vi "메인.vi"() -> ()   [LabVIEW 2021]
uses:
  ctl/AI.ctl
  ctl/RS232.ctl
  ctl/DB.ctl
  ctl/sm.ctl
  ctl/CNN.ctl
  <vilib>/userDefined/High Color/IMAQdx.ctl
  <vilib>/Utility/sysdir.llb/System Directory Type.ctl
  <vilib>/DAQmx/read.llb/DAQmx Read (Analog 1D Wfm NChan NSamp).vi
  <vilib>/Analysis/baseanly.llb/Mean (DBL).vi
  <vilib>/Utility/file.llb/Write Delimited Spreadsheet (DBL).vi
  <vilib>/addons/database/Connection.llb/DB Tools Open Connec (String).vi
  <vilib>/Instr/_visa.llb/VISA Configure Serial Port (Instr).vi
  <vilib>/DAQmx/create/channels.llb/DAQmx Create Channel (AI-Voltage-Basic).vi
  <vilib>/DAQmx/configure/timing.llb/DAQmx Timing (Sample Clock).vi
  <vilib>/DAQmx/miscellaneous.llb/DAQmx Fill In Error Info.vi
  <vilib>/Analysis/NI_AALBase.lvlib
  <vilib>/vision/driver/NI_Vision_Acquisition_Software.lvlib
  <vilib>/addons/database/NI_Database_API.lvlib
panel:
  out "CNN Result":string[](array[string])
  out "Factory 상태":string
  in  "여러 열 리스트박스 2":i32(listbox)
  in  "여러 열 리스트박스":i32(listbox)
  out "Image":T1(plugin-control)
  out "온도":u32[](array[numeric])
  out "배열":dbl[](array[numeric])
  out "거리 센서":waveform(dbl)(graph)
  out "기울기 그래프":waveform(dbl)[](graph)
  out "가속도 그래프":waveform(dbl)(graph)
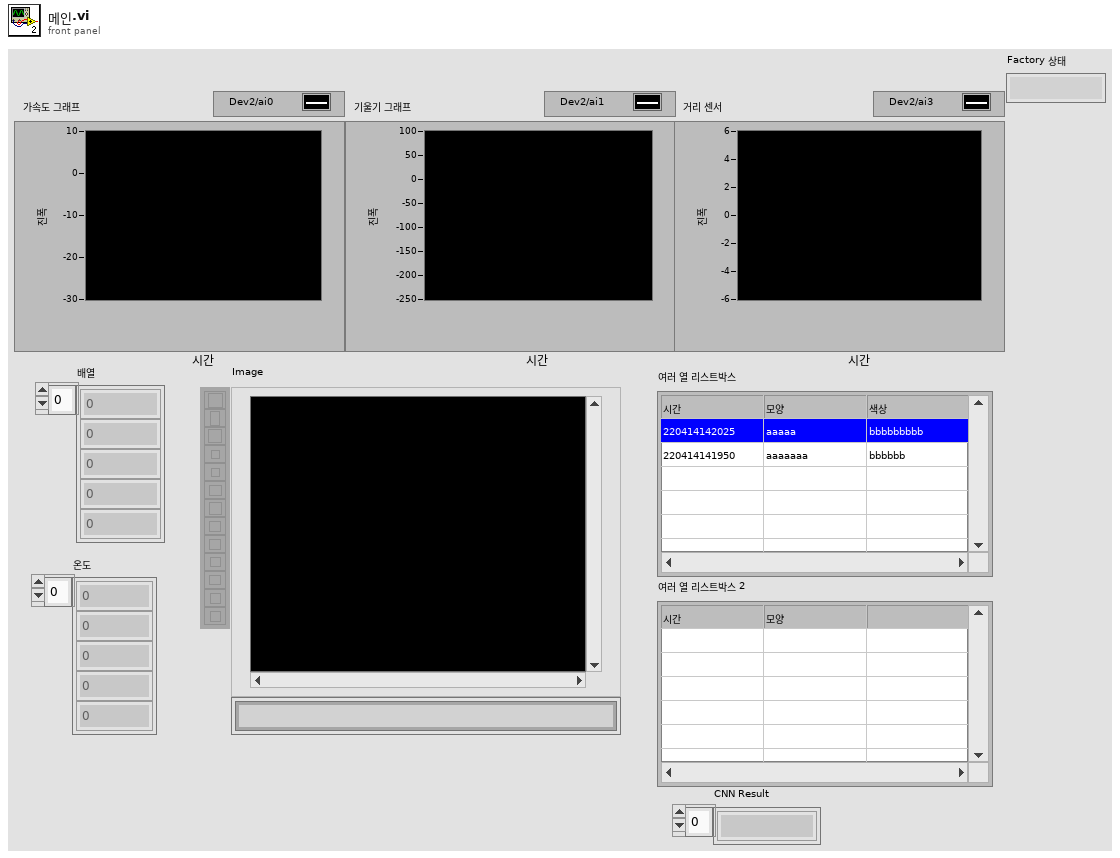
[diagram p1: front panel]
types:
  T1 = typedef "IMAQ Image.ctl" = refnum<image>
  T2 = typedef "비전.ctl" = cluster{"상태":enum16{"초기화", "설정", "상시읽기", "트리거읽기", "닫기", "프로그램정지"}, "값":variant}
  T3 = typedef "CNN.ctl" = cluster{"상태":enum16{"CNN 통신", "프로그램정지"}, "값":variant}
  T4 = typedef "sm.ctl" = cluster{"상태":enum16{"SM통신", "프로그램정지"}, "값":variant}
  T5 = cluster{"메인":refnum<queue>, "AI":refnum<queue>, "RS-232":refnum<queue>, "SM":refnum<queue>, "CNN":refnum<queue>, "DB":refnum<queue>, "비전":refnum<queue>}
  T6 = typedef "메인.ctl" = cluster{"상태":enum16{"초기화", "프로그램정지"}, "값":variant}
  T7 = typedef "DB.ctl" = cluster{"상태":enum16{"초기화", "설정", "값 쓰기", "에러 쓰기", "닫기", "프로그램 정지"}, "값":variant}
  T8 = typedef "RS232.ctl" = cluster{"상태":enum16{"초기화", "설정", "읽기", "닫기", "프로그램정지"}, "값":variant}
  T9 = typedef "AI.ctl" = cluster{"상태":enum16{"초기화", "설정", "읽기", "닫기", "프로그램정지"}, "값":variant}
  T10 = enum16{"초기화", "설정", "값 쓰기", "에러 쓰기", "닫기", "프로그램 정지"}
  T11 = typedef "NI_Database_API.lvlib/Conn ObjectReference.ctl" = refnum<k1>
  T12 = cluster{"[0]":string, "[1]":string, "[2]":string}
  T13 = typedef "IMAQdx.ctl" = refnum<k21>
  T14 = enum16{"초기화", "설정", "상시읽기", "트리거읽기", "닫기", "프로그램정지"}
  T15 = typedef "System Directory Type.ctl" = i32
  T16 = enum16{"Standard", "Buffered", "CRLF", "Immediate"}
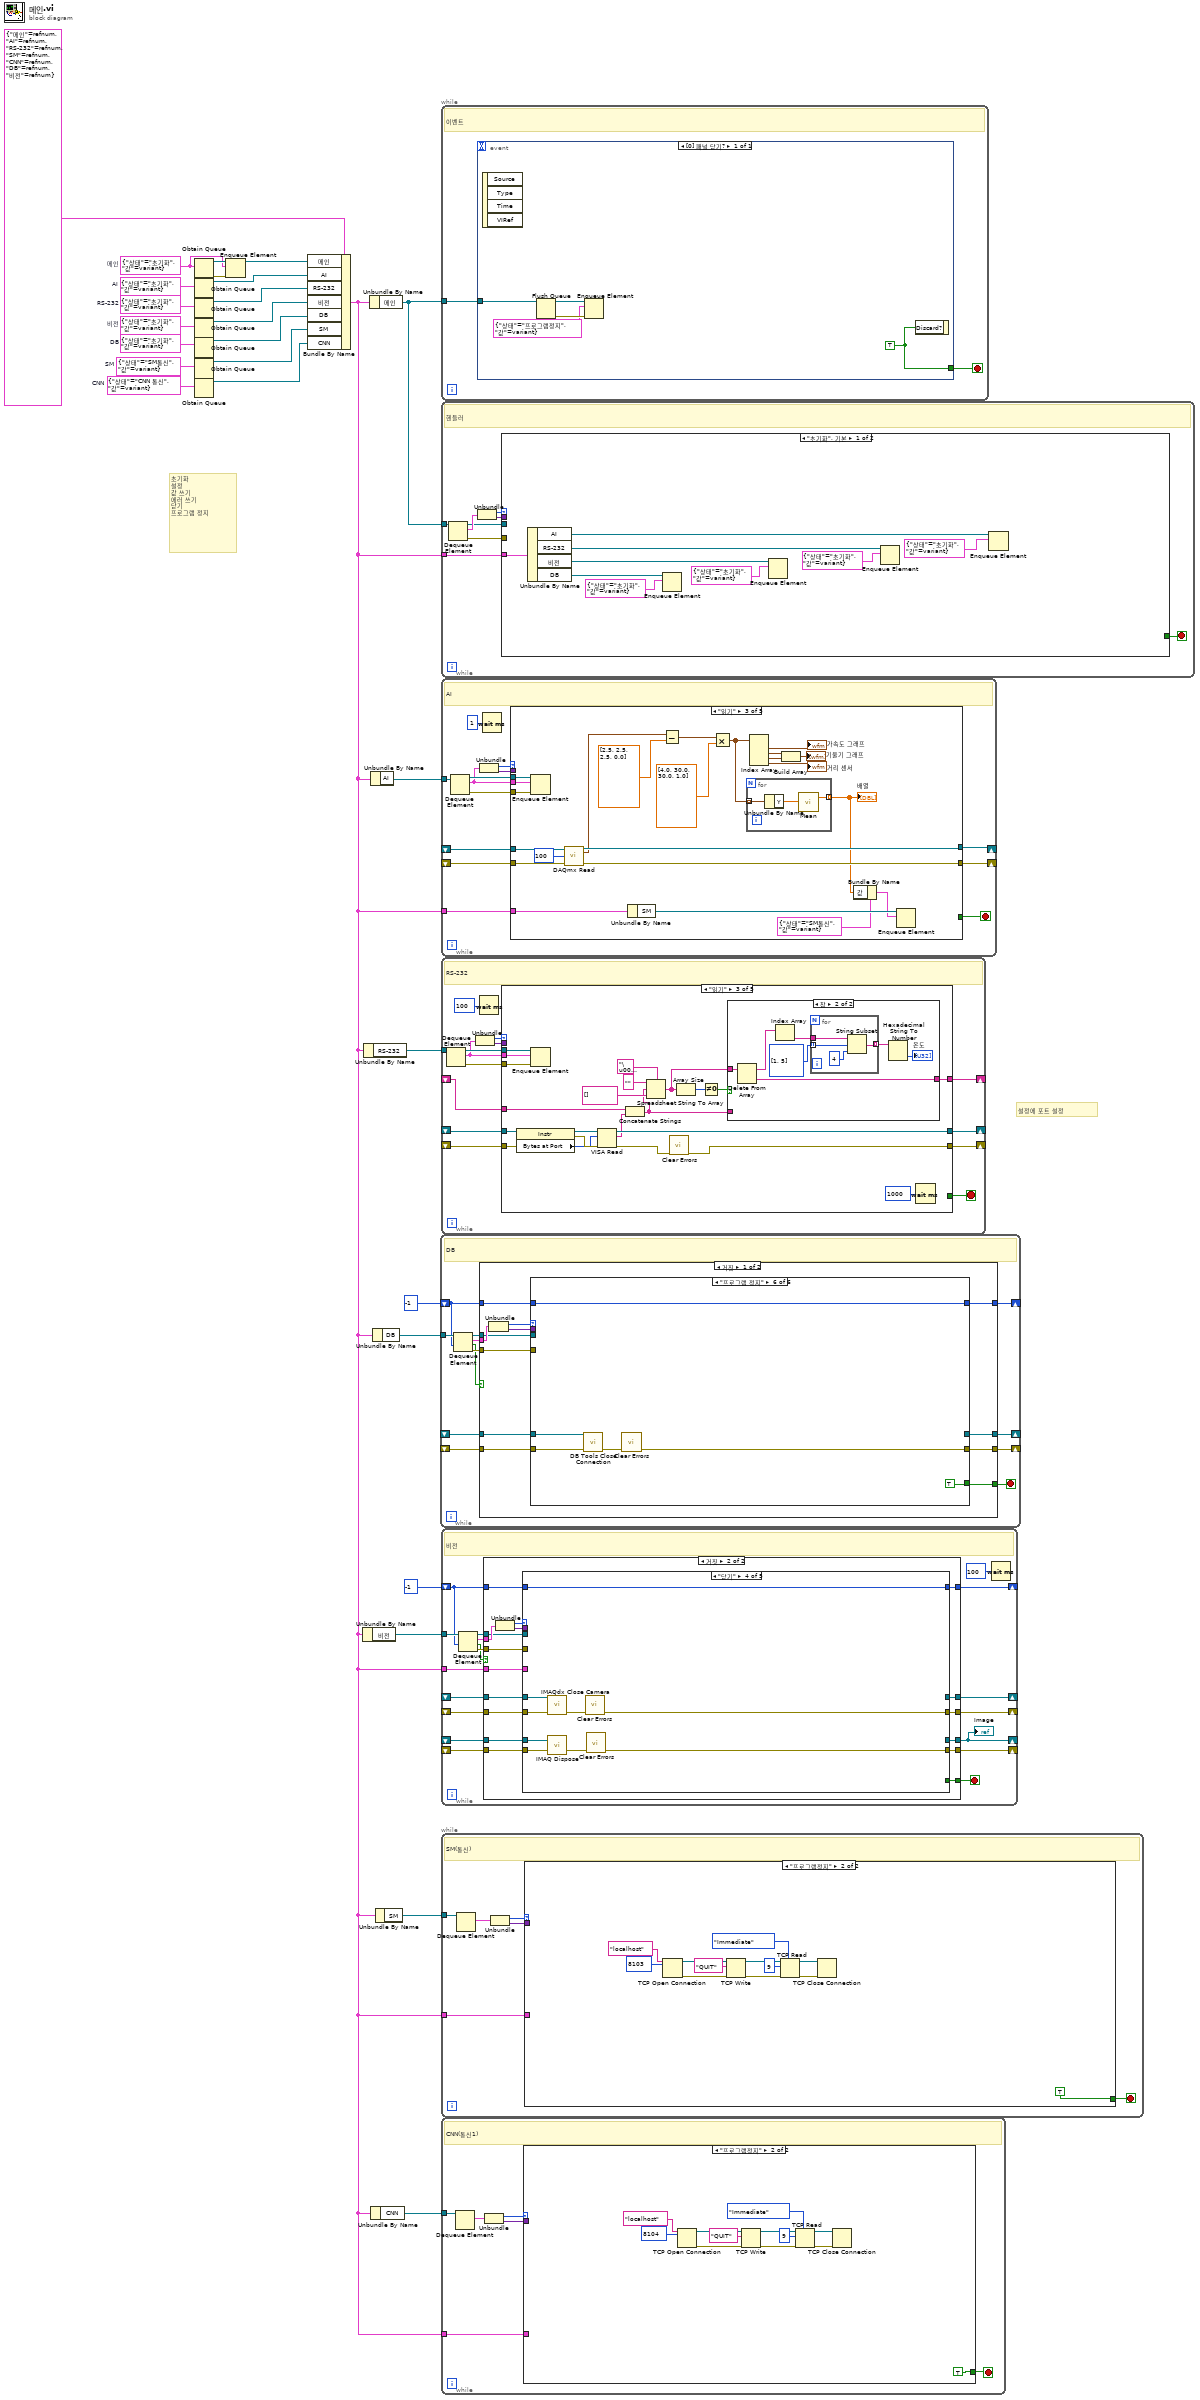
[diagram p0: block diagram]
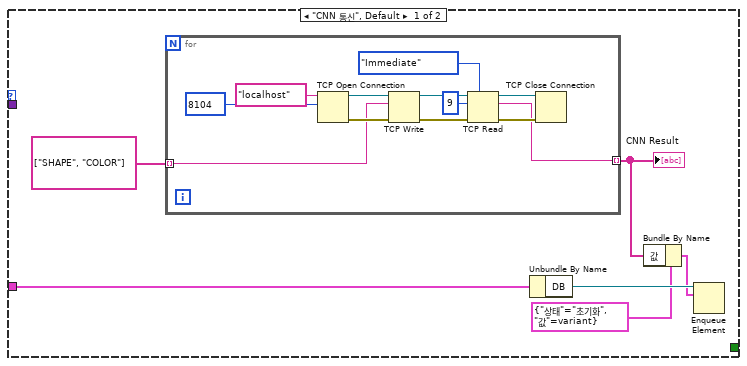
[diagram p2: hidden frame]
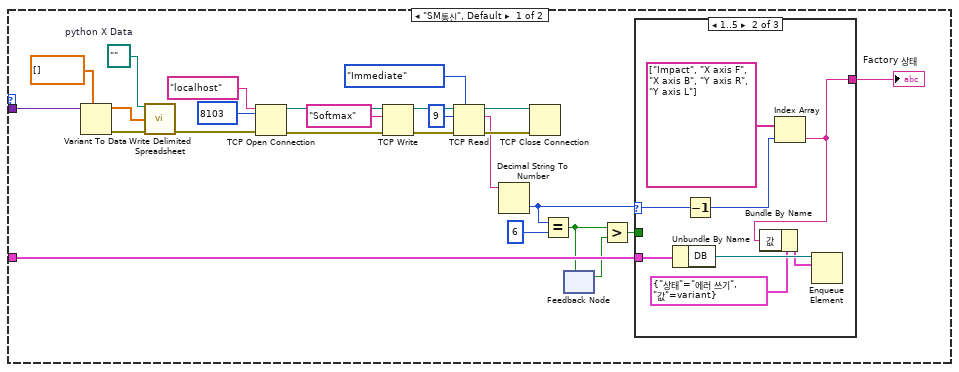
[diagram p3: hidden frame]
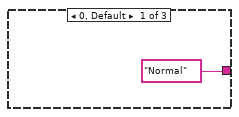
[diagram p4: hidden frame]
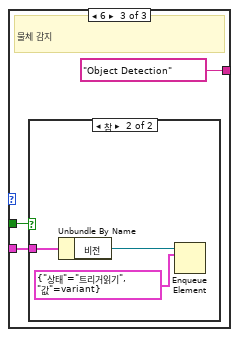
[diagram p5: hidden frame]
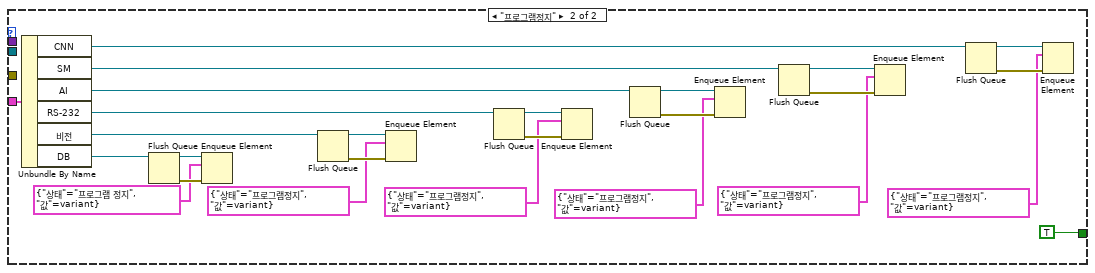
[diagram p7: hidden frame]
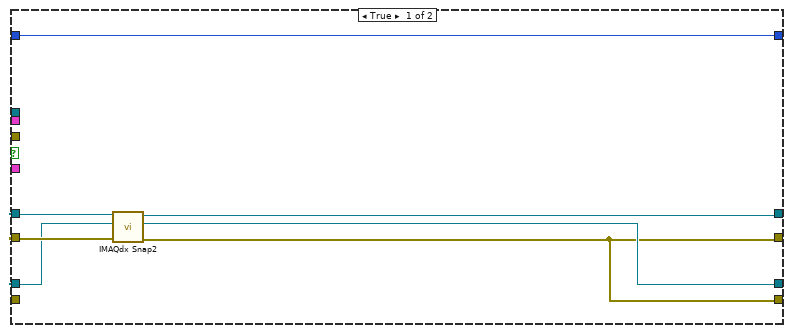
[diagram p8: hidden frame]
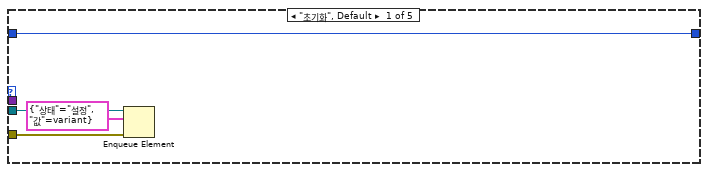
[diagram p9: hidden frame]
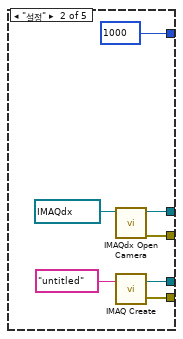
[diagram p10: hidden frame]
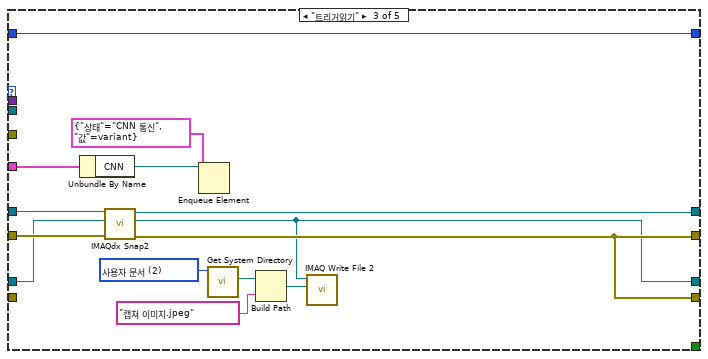
[diagram p11: hidden frame]
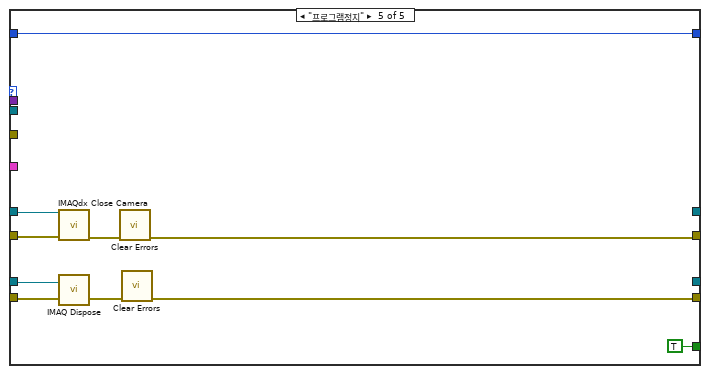
[diagram p12: hidden frame]
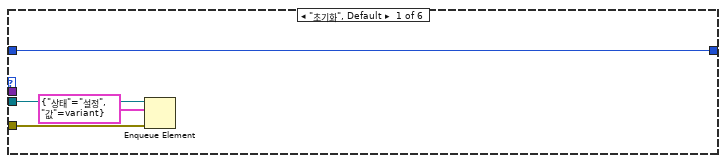
[diagram p13: hidden frame]
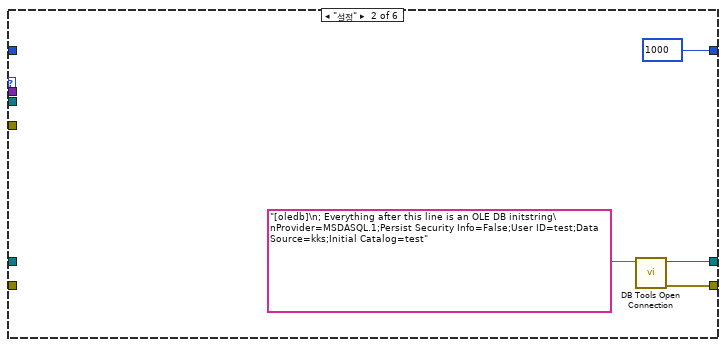
[diagram p14: hidden frame]
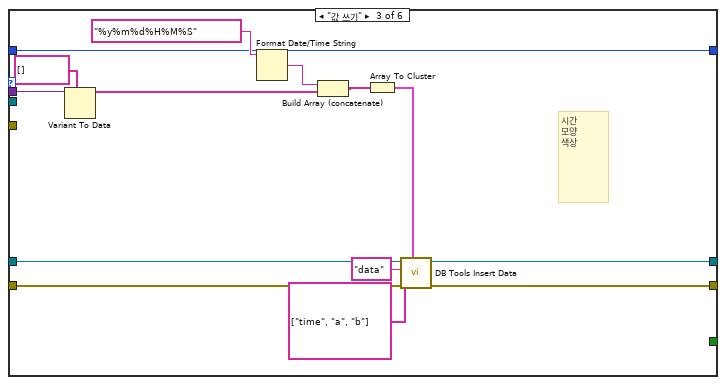
[diagram p15: hidden frame]
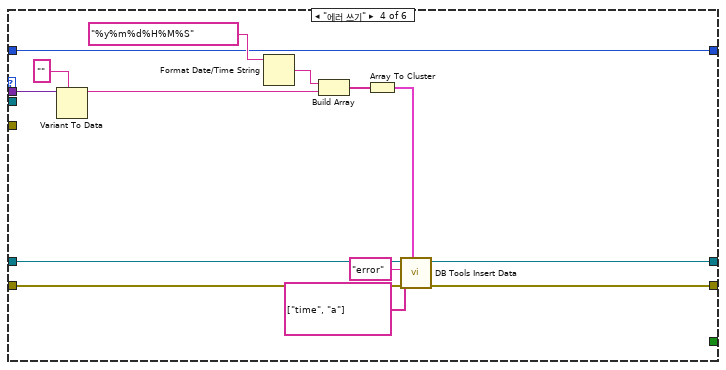
[diagram p16: hidden frame]
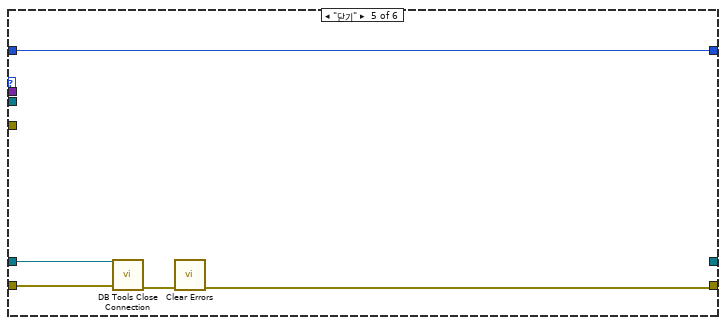
[diagram p17: hidden frame]
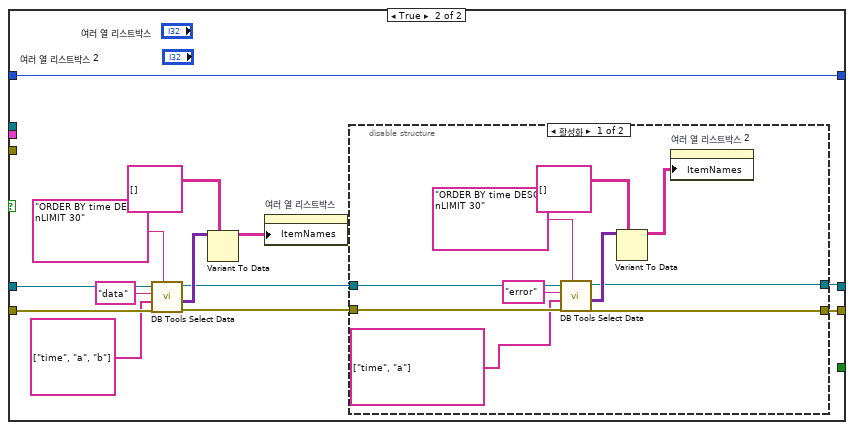
[diagram p18: hidden frame]
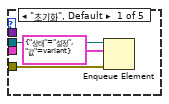
[diagram p20: hidden frame]
diagram:
  w2 = T2 {"상태"=enum."초기화", "값"=variant}  # 비전
  w9 = T3 {"상태"=enum."CNN 통신", "값"=variant}  # CNN
  w10 = T4 {"상태"=enum."SM통신", "값"=variant}  # SM
  w18 = T6 {"상태"=enum."초기화", "값"=variant}  # 메인
  w25 = T7 {"상태"=enum."초기화", "값"=variant}  # DB
  w26 = T8 {"상태"=enum."초기화", "값"=variant}  # RS-232
  w27 = T9 {"상태"=enum."초기화", "값"=variant}  # AI
  # "초기화\n설정\n값 쓰기\n에러 쓰기\n닫기\n프로그램 정지"
  # "설정에 포트 설정"
  n1 = Obtain Queue(element data type=w18) -> (queue out=w23:refnum<queue>, error out=w19:errorcluster)  [unwired: 4 in, 1 out]
  n2 = Obtain Queue(element data type=w27) -> (queue out=w22:refnum<queue>)  [unwired: 4 in, 2 out]
  n3 = Obtain Queue(element data type=w26) -> (queue out=w21:refnum<queue>)  [unwired: 4 in, 2 out]
  n4 = Obtain Queue(element data type=w2) -> (queue out=w1:refnum<queue>)  [unwired: 4 in, 2 out]
  n5 = Obtain Queue(element data type=w25) -> (queue out=w3:refnum<queue>)  [unwired: 4 in, 2 out]
  n6 = Obtain Queue(element data type=w10) -> (queue out=w8:refnum<queue>)  [unwired: 4 in, 2 out]
  n7 = Obtain Queue(element data type=w9) -> (queue out=w7:refnum<queue>)  [unwired: 4 in, 2 out]
  n8 = Enqueue Element(queue=w23, element=w18, error in (no error)=w19) -> (queue out=w20:refnum<queue>)  [unwired: 1 in, 2 out]
  n9 = Bundle By Name(cluster=T5 {"메인"=refnum, "AI"=refnum, "RS-232"=refnum, "SM"=refnum, "CNN"=refnum, "DB"=refnum, "비전"=refnum}, "메인"=w20, "AI"=w22, "RS-232"=w21, "비전"=w1, "DB"=w3, "SM"=w8, "CNN"=w7) -> (w4:T5)
  n10 = Unbundle By Name(w4) -> ("비전"=w13:refnum<queue>)
  n11 = Unbundle By Name(w4) -> ("RS-232"=w15:refnum<queue>)
  n12 = Unbundle By Name(w4) -> ("메인"=w17:refnum<queue>)
  n13 = Unbundle By Name(w4) -> ("AI"=w16:refnum<queue>)
  n14 = Unbundle By Name(w4) -> ("CNN"=w5:refnum<queue>)
  n15 = Unbundle By Name(w4) -> ("DB"=w14:refnum<queue>)
  n16 = Unbundle By Name(w4) -> ("SM"=w6:refnum<queue>)
  n17 = while {
    tunnel: w14 -> [w38]
    shift-right: [w34] -> _
    shift-left: _ -> [w32]
    shift-right: [w33] -> _
    shift-left: _ -> [w31]
    shift-right: [w30] -> _
    shift-left: -1 -> [w29]
    stop <- w35 stop-if-true
    # "DB"
    n18 = Dequeue Element(queue=w38, timeout in ms (-1)=w29) -> (queue out=w37:refnum<queue>, element=w39:T7, timed out?=w28:bool, error out=w36:errorcluster)  [unwired: 1 in]
    n19 = case shown="거짓" w28 {
      tunnel: w39 -> [w51 _]
      tunnel: w37 -> [w49 _]
      tunnel: w36 -> [w48 _]
      tunnel: [w47 _] -> w35
      tunnel: [w46 w102] -> w34
      tunnel: [w45 w99] -> w33
      tunnel: w32 -> [w44 w110]
      tunnel: w31 -> [w43 w109]
      tunnel: [w42 w111] -> w30
      tunnel: w29 -> [w41 w111]
      frame False {
        n20 = Unbundle(w51) -> ("상태"=w40:T10, "값"=w50:variant)
        n21 = case shown="\"프로그램 정지\"" w40 {
          tunnel: w50 -> [_ _ w69 w83 _ _]
          tunnel: w49 -> [w55 _ _ _ _ _]
          tunnel: w48 -> [w54 _ _ _ _ _]
          tunnel: [_ _ _ _ _ TRUE] -> w47
          tunnel: [_ w58 w71 w85 _ _] -> w46
          tunnel: [_ w57 w70 w84 w89 w94] -> w45
          tunnel: w44 -> [_ _ w73 w87 w92 w96]
          tunnel: w43 -> [_ _ w72 w86 w91 w95]
          tunnel: [w53 1000 w60 w74 w88 w93] -> w42
          tunnel: w41 -> [w53 _ w60 w74 w88 w93]
          frame "초기화", Default {
            n22 = Enqueue Element(queue=w55, element=T7 {"상태"=enum."설정", "값"=variant} ("원소"), error in (no error)=w54) -> ()  [unwired: 1 in, 3 out]
          }
          frame "설정" {
            n23 = call-poly <vilib>:"DB Tools Open Connection.vi"("connection information"="[oledb]\n; Everything after this line is an OLE DB initstring\nProvider=MSDASQL.1;Persist Security Info=False;User ID=test;Data Source=kks;Initial Catalog=test") -> ("error out"=w57:errorcluster, "connection reference"=w58:T11)  [unwired: 7 in]
          }
          frame "값 쓰기" {
            # "시간\n모양\n색상"
            n24 = Variant To Data(type=string[] [], Variant=w69) -> (data=w65:string[])  [unwired: 1 in, 1 out]
            n25 = Format Date/Time String(time format string (%c)="%y%m%d%H%M%S" ("시간 포맷 문자열 (%c)")) -> (date/time string=w64:string)  [unwired: 2 in]
            n26 = Build Array (concatenate)(w64, w65) -> (w63:string[])
            n27 = Array To Cluster(array=w63) -> (cluster=w67:T12)
            n28 = call <vilib>:"DB Tools Insert Data.vi"("data"=w67, "error in (no error)"=w72, "columns"=string[] ["time", "a", "b"], "table"="data", "connection reference"=w73) -> ("error out"=w70:errorcluster, "connection reference out"=w71:T11)  [unwired: 5 in]
          }
          frame "에러 쓰기" {
            # "가속도, 기울기 X, 기울기 Y, 거리, 온도1, 온도2"
            n29 = Variant To Data(type="", Variant=w83) -> (data=w77:string)  [unwired: 1 in, 1 out]
            n30 = Format Date/Time String(time format string (%c)="%y%m%d%H%M%S" ("시간 포맷 문자열 (%c)")) -> (date/time string=w79:string)  [unwired: 2 in]
            n31 = Build Array(w79, w77) -> (w80:string[])
            n32 = Array To Cluster(array=w80) -> (cluster=w82:cluster{"[0]":string, "[1]":string})
            n33 = call <vilib>:"DB Tools Insert Data.vi"("data"=w82, "error in (no error)"=w86, "columns"=string[] ["time", "a"], "table"="error", "connection reference"=w87) -> ("error out"=w84:errorcluster, "connection reference out"=w85:T11)  [unwired: 5 in]
          }
          frame "닫기" {
            n34 = call <vilib>:"DB Tools Close Connection.vi"("error in (no error)"=w91, "connection reference"=w92) -> ("error out"=w90:errorcluster)  [unwired: 5 in]
            n35 = call <vilib>:"Clear Errors.vi"("error in (no error)"=w90) -> ("error out"=w89:errorcluster)  [unwired: 5 in, 1 out]
          }
          frame "프로그램 정지" {
            n36 = call <vilib>:"DB Tools Close Connection.vi"("error in (no error)"=w95, "connection reference"=w96) -> ("error out"=w97:errorcluster)  [unwired: 5 in]
            n37 = call <vilib>:"Clear Errors.vi"("error in (no error)"=w97) -> ("error out"=w94:errorcluster)  [unwired: 5 in, 1 out]
          }
        }
      }
      frame True {
        n38 = call <vilib>:"DB Tools Select Data.vi"("condition"="ORDER BY time DESC\nLIMIT 30", "error in (no error)"=w109, "columns"=string[] ["time", "a", "b"], "table"="data", "connection reference"=w110) -> ("error out"=w100:errorcluster, "data"=w105:variant[][], "connection reference out"=w103:T11)  [unwired: 1 in]
        n39 = Variant To Data(type=string[][] [], Variant=w105) -> (data=w104:string[][])  [unwired: 1 in, 1 out]
        n40 = property on="여러 열 리스트박스" class="MCListbox (엄격한)"("ItemNames"=w104) -> ()  [unwired: 2 in, 2 out]
        n41 = disable-structure shown="활성화" {
          disable-tunnel: w103 -> [w118 w122]
          disable-tunnel: w100 -> [w117 _]
          disable-tunnel: [w116 w122] -> w102
          disable-tunnel: [w115 _] -> w99
          frame Enabled {
            n42 = call <vilib>:"DB Tools Select Data.vi"("condition"="ORDER BY time DESC\nLIMIT 30", "error in (no error)"=w117, "columns"=string[] ["time", "a"] ("String"), "table"="error", "connection reference"=w118) -> ("error out"=w115:errorcluster, "data"=w121:variant[][], "connection reference out"=w116:T11)  [unwired: 1 in]
            n43 = Variant To Data(type=string[][] [], Variant=w121) -> (data=w113:string[][])  [unwired: 1 in, 1 out]
            n44 = property on="여러 열 리스트박스 2" class="MCListbox (엄격한)"("ItemNames"=w113) -> ()  [unwired: 2 in, 2 out]
          }
          frame Disabled {
          }
        }
      }
    }
  }
  n45 = while {
    tunnel: w17 -> [w123]
    stop <- w124 stop-if-true
    # "이벤트"
    n46 = event shown="[0] 패널 닫기?" {
      selector: _ -> [_]
      dyn-events: _ -> [_]
      timeout: _ -> [_]
      tunnel: [w129] -> w124
      tunnel: w123 -> [w126]
      event Panel Close? {
        w129 = TRUE ("버림?")
        n47 = event-data() -> ()  [unwired: 1 in, 4 out]
        n48 = Flush Queue(queue=w126) -> (queue out=w127:refnum<queue>, error out=w128:errorcluster)  [unwired: 1 in, 1 out]
        n49 = Enqueue Element(queue=w127, element=T6 {"상태"=enum."프로그램정지", "값"=variant} ("원소"), error in (no error)=w128) -> ()  [unwired: 1 in, 3 out]
        n50 = event-data("Discard?"=w129) -> ()  [unwired: 1 in, 1 out]
      }
    }
  }
  n51 = while {
    tunnel: w4 -> [w137]
    tunnel: w17 -> [w136]
    stop <- w130 stop-if-true
    # "헨들러"
    n52 = Dequeue Element(queue=w136) -> (queue out=w134:refnum<queue>, element=w135:T6, error out=w131:errorcluster)  [unwired: 2 in, 1 out]
    n53 = Unbundle(w135) -> ("상태"=w133:enum16{"초기화", "프로그램정지"}, "값"=w132:variant)
    n54 = case shown="\"초기화\", 기본" w133 {
      tunnel: w137 -> [w144 w158]
      tunnel: w134 -> [_ _]
      tunnel: w132 -> [_ _]
      tunnel: w131 -> [_ _]
      tunnel: [_ TRUE] -> w130
      frame "초기화", Default {
        n55 = Unbundle By Name(w144) -> ("AI"=w143:refnum<queue>, "RS-232"=w142:refnum<queue>, "비전"=w141:refnum<queue>, "DB"=w140:refnum<queue>)
        n56 = Enqueue Element(queue=w140, element=T7 {"상태"=enum."초기화", "값"=variant} ("원소")) -> ()  [unwired: 2 in, 3 out]
        n57 = Enqueue Element(queue=w141, element=T2 {"상태"=enum."초기화", "값"=variant} ("원소")) -> ()  [unwired: 2 in, 3 out]
        n58 = Enqueue Element(queue=w142, element=T8 {"상태"=enum."초기화", "값"=variant} ("원소")) -> ()  [unwired: 2 in, 3 out]
        n59 = Enqueue Element(queue=w143, element=T9 {"상태"=enum."초기화", "값"=variant} ("원소")) -> ()  [unwired: 2 in, 3 out]
      }
      frame "프로그램정지" {
        n60 = Unbundle By Name(w158) -> ("CNN"=w151:refnum<queue>, "SM"=w152:refnum<queue>, "AI"=w165:refnum<queue>, "RS-232"=w166:refnum<queue>, "비전"=w172:refnum<queue>, "DB"=w171:refnum<queue>)
        n61 = Flush Queue(queue=w171) -> (queue out=w168:refnum<queue>, error out=w167:errorcluster)  [unwired: 1 in, 1 out]
        n62 = Enqueue Element(queue=w168, element=T7 {"상태"=enum."프로그램 정지", "값"=variant} ("원소"), error in (no error)=w167) -> ()  [unwired: 1 in, 3 out]
        n63 = Flush Queue(queue=w172) -> (queue out=w169:refnum<queue>, error out=w170:errorcluster)  [unwired: 1 in, 1 out]
        n64 = Enqueue Element(queue=w169, element=T2 {"상태"=enum."프로그램정지", "값"=variant} ("원소"), error in (no error)=w170) -> ()  [unwired: 1 in, 3 out]
        n65 = Flush Queue(queue=w166) -> (queue out=w163:refnum<queue>, error out=w164:errorcluster)  [unwired: 1 in, 1 out]
        n66 = Enqueue Element(queue=w163, element=T8 {"상태"=enum."프로그램정지", "값"=variant} ("원소"), error in (no error)=w164) -> ()  [unwired: 1 in, 3 out]
        n67 = Flush Queue(queue=w165) -> (queue out=w162:refnum<queue>, error out=w161:errorcluster)  [unwired: 1 in, 1 out]
        n68 = Enqueue Element(queue=w162, element=T9 {"상태"=enum."프로그램정지", "값"=variant} ("원소"), error in (no error)=w161) -> ()  [unwired: 1 in, 3 out]
        n69 = Flush Queue(queue=w152) -> (queue out=w154:refnum<queue>, error out=w153:errorcluster)  [unwired: 1 in, 1 out]
        n70 = Enqueue Element(queue=w154, element=T4 {"상태"=enum."프로그램정지", "값"=variant} ("원소"), error in (no error)=w153) -> ()  [unwired: 1 in, 3 out]
        n71 = Flush Queue(queue=w151) -> (queue out=w155:refnum<queue>, error out=w156:errorcluster)  [unwired: 1 in, 1 out]
        n72 = Enqueue Element(queue=w155, element=T3 {"상태"=enum."프로그램정지", "값"=variant} ("원소"), error in (no error)=w156) -> ()  [unwired: 1 in, 3 out]
      }
    }
  }
  n73 = while {
    tunnel: w16 -> [w185]
    shift-right: [w179] -> _
    shift-left: _ -> [w177]
    shift-right: [w178] -> _
    shift-left: _ -> [w176]
    tunnel: w4 -> [w173]
    stop <- w181 stop-if-true
    # "AI"
    n74 = Dequeue Element(queue=w185) -> (queue out=w183:refnum<queue>, element=w174:T9, error out=w182:errorcluster)  [unwired: 2 in, 1 out]
    n75 = Unbundle(w174) -> ("상태"=w184:enum16{"초기화", "설정", "읽기", "닫기", "프로그램정지"}, "값"=w180:variant)
    n76 = Wait (ms)(milliseconds to wait=u32 1 ("대기 시간 (ms)")) -> ()  [unwired: 1 out]
    n77 = case shown="\"읽기\"" w184 {
      tunnel: w183 -> [w188 w192 w210 _ _]
      tunnel: w182 -> [w187 w191 w209 _ _]
      tunnel: [_ _ _ _ TRUE] -> w181
      tunnel: w180 -> [_ _ _ _ _]
      tunnel: [_ w198 w222 _ _] -> w179
      tunnel: [errorcluster {"status"=FALSE, "code"=0, "source"=""} ("error out") w197 w221 w229 w233] -> w178
      tunnel: w177 -> [_ _ w225 w232 w235]
      tunnel: w176 -> [_ _ w224 w231 w234]
      tunnel: w174 -> [_ _ w208 _ _]
      tunnel: w173 -> [_ _ w207 _ _]
      frame "초기화", Default {
        n78 = Enqueue Element(queue=w188, element=T9 {"상태"=enum."설정", "값"=variant} ("원소"), error in (no error)=w187) -> ()  [unwired: 1 in, 3 out]
      }
      frame "설정" {
        w194 = 10123 items=["유한 샘플"=10178, "연속 샘플"=10123, "하드웨어 타이밍에 의한 단일 포인트"=12522] ("sample mode")
        w195 = 10106 items=["기본"=-1, "RSE"=10083, "NRSE"=10078, "차동"=10106, "유사 차동"=12529] ("input terminal configuration")
        n79 = Enqueue Element(queue=w192, element=T9 {"상태"=enum."읽기", "값"=variant} ("원소"), error in (no error)=w191) -> ()  [unwired: 1 in, 3 out]
        n80 = call-poly <vilib>:"DAQmx Create Virtual Channel.vi"("input terminal configuration"=w195, "physical channels"=tag "Dev2/ai0:3") -> ("task out"=w202:refnum<k21>, "error out"=w201:errorcluster)  [unwired: 12 in]
        n81 = call-poly <vilib>:"DAQmx Timing.vi"("task/channels in"=w202, "sample mode"=w194, "rate"=1000.0, "error in"=w201) -> ("task out"=w200:refnum<k21>, "error out"=w199:errorcluster)  [unwired: 10 in]
        n82 = call <vilib>:"DAQmx Start Task.vi"("task/channels in"=w200, "error in"=w199) -> ("task out"=w198:refnum<k21>, "error out"=w197:errorcluster)  [unwired: 12 in]
      }
      frame "읽기" {
        n83 = Enqueue Element(queue=w210, element=w208, error in (no error)=w209) -> ()  [unwired: 1 in, 3 out]
        n84 = call-poly <vilib>:"DAQmx Read.vi"("task/channels in"=w225, "number of samples per channel"=100, "error in"=w224) -> ("task out"=w222:refnum<k21>, "data"=w219:waveform(dbl)[], "error out"=w221:errorcluster)  [unwired: 10 in]
        n85 = Unbundle By Name(w207) -> ("SM"=w206:refnum<queue>)
        n86 = Subtract(x=w219, y=dbl[] [2.5, 2.5, 2.5, 0.0]) -> (x-y=w218:waveform(dbl)[])
        n87 = Multiply(x=w218, y=dbl[] [4.0, 30.0, 30.0, 1.0]) -> (x*y=w211:waveform(dbl)[])
        n88 = for {
          tunnel: w211 -> [w228] mode=indexing
          tunnel: [w226] -> w205 mode=indexing
          n89 = Unbundle By Name(w228) -> ("Y"=w227:dbl[])
          n90 = call-poly <vilib>:"Mean.vi"("X"=w227) -> ("mean"=w226:dbl)  [unwired: 1 out]
        }
        "배열" <- w205
        n91 = Index Array(array=w211) -> (element #1=→"가속도 그래프":waveform(dbl), element #2=w216:waveform(dbl), element #3=w215:waveform(dbl), element #4=→"거리 센서":waveform(dbl))  [unwired: 4 in]
        n92 = Build Array(w216, w215) -> (→"기울기 그래프":waveform(dbl)[])
        n93 = Bundle By Name(cluster=T4 {"상태"=enum."SM통신", "값"=variant} ("원소"), "값"=w205) -> (w203:T4)
        n94 = Enqueue Element(queue=w206, element=w203) -> ()  [unwired: 2 in, 3 out]
      }
      frame "닫기" {
        n95 = call <vilib>:"DAQmx Stop Task.vi"("task/channels in"=w232, "error in"=w231) -> ("error out"=w230:errorcluster)  [unwired: 12 in, 1 out]
        n96 = call <vilib>:"Clear Errors.vi"("error in (no error)"=w230) -> ("error out"=w229:errorcluster)  [unwired: 5 in, 1 out]
      }
      frame "프로그램정지" {
        n97 = call <vilib>:"DAQmx Stop Task.vi"("task/channels in"=w235, "error in"=w234) -> ("error out"=w236:errorcluster)  [unwired: 12 in, 1 out]
        n98 = call <vilib>:"Clear Errors.vi"("error in (no error)"=w236) -> ("error out"=w233:errorcluster)  [unwired: 5 in, 1 out]
      }
    }
  }
  n99 = while {
    tunnel: w15 -> [w251]
    shift-right: [w245] -> _
    shift-left: _ -> [w243]
    shift-right: [w244] -> _
    shift-left: _ -> [w242]
    shift-right: [w240] -> _
    shift-left: _ -> [w239]
    stop <- w246 stop-if-true
    # "RS-232"
    n100 = Dequeue Element(queue=w251) -> (queue out=w248:refnum<queue>, element=w241:T8, error out=w247:errorcluster)  [unwired: 2 in, 1 out]
    n101 = Unbundle(w241) -> ("상태"=w250:enum16{"초기화", "설정", "읽기", "닫기", "프로그램정지"}, "값"=w249:variant)
    n102 = Wait (ms)(milliseconds to wait=u32 100 ("대기 시간 (ms)")) -> ()  [unwired: 1 out]
    n103 = case shown="\"읽기\"" w250 {
      tunnel: w249 -> [_ _ _ _ _]
      tunnel: w248 -> [w254 w257 w277 _ _]
      tunnel: w247 -> [w253 w256 w276 _ _]
      tunnel: [_ _ _ _ TRUE] -> w246
      tunnel: [_ w260 w284 _ _] -> w245
      tunnel: [_ w259 w263 w297 w301] -> w244
      tunnel: w243 -> [_ _ w282 w300 w303]
      tunnel: w242 -> [_ _ w280 w299 w302]
      tunnel: w241 -> [_ _ w275 _ _]
      tunnel: [_ _ w267 _ _] -> w240
      tunnel: w239 -> [_ _ w266 _ _]
      frame "초기화", Default {
        n104 = Enqueue Element(queue=w254, element=T8 {"상태"=enum."설정", "값"=variant} ("원소"), error in (no error)=w253) -> ()  [unwired: 1 in, 3 out]
      }
      frame "설정" {
        n105 = Enqueue Element(queue=w257, element=T8 {"상태"=enum."읽기", "값"=variant} ("원소"), error in (no error)=w256) -> ()  [unwired: 1 in, 3 out]
        n106 = call-poly "VISA Configure Serial Port"("VISA resource name"=refnum<visa-resource-name> "COM3") -> ("VISA resource name out"=w262:refnum<visa-resource-name>, "error out"=w261:errorcluster)  [unwired: 13 in]
        n107 = VISA Flush I/O Buffer(VISA resource name=w262, error in (no error)=w261) -> (VISA resource name out=w260:refnum<visa-resource-name>, error out=w259:errorcluster)  [unwired: 1 in]
      }
      frame "읽기" {
        n108 = property class="Instr"(reference=w282, error in=w280) -> (reference out=w281:refnum<visa-resource-name>, error out=w279:errorcluster, "Bytes at Port"=w278:u32)
        n109 = Enqueue Element(queue=w277, element=w275, error in (no error)=w276) -> ()  [unwired: 1 in, 3 out]
        n110 = VISA Read(VISA resource name=w281, byte count=w278, error in (no error)=w279) -> (VISA resource name out=w284:refnum<visa-resource-name>, read buffer=w265:string, error out=w283:errorcluster)  [unwired: 1 out]
        n111 = Concatenate Strings(w266, w265) -> (w264:string)
        n112 = Spreadsheet String To Array(delimiter (Tab)="\u0004" ("구분 문자 (탭)"), format string="" ("포맷 문자열"), spreadsheet string=w264, array type (2D Dbl)=string[] []) -> (array=w268:string[])
        n113 = call <vilib>:"Clear Errors.vi"("error in (no error)"=w283) -> ("error out"=w263:errorcluster)  [unwired: 5 in, 1 out]
        n114 = Array Size(array=w268) -> (size(s)=w270:i32)
        n115 = Not Equal To 0?(x=w270) -> (x != 0?=w269:bool)
        n116 = case shown="참" w269 {
          tunnel: w268 -> [_ w292]
          tunnel: [w285 w291] -> w267
          tunnel: w264 -> [w285 _]
          frame False {
          }
          frame True {
            n117 = Delete From Array(array=w292) -> (deleted portion=w291:string, array with subset deleted=w290:string[])  [unwired: 2 in]
            n118 = Index Array(array=w290) -> (element=w289:string)  [unwired: 1 in]
            n119 = for {
              tunnel: w289 -> [w296]
              tunnel: i32[] [1, 5] ("오프셋(0)") -> [w294] mode=indexing
              tunnel: [w293] -> w286 mode=indexing
              n120 = String Subset(string=w296, offset (0)=w294, length (rest)=4 ("길이(나머지)")) -> (substring=w293:string)
            }
            n121 = Hexadecimal String To Number(string=w286) -> (number=→"온도":u32[])  [unwired: 2 in, 1 out]
          }
        }
        n122 = Wait (ms)(milliseconds to wait=u32 1000 ("대기 시간 (ms)")) -> ()  [unwired: 1 out]
      }
      frame "닫기" {
        n123 = VISA Close(VISA resource name=w300, error in (no error)=w299) -> (error out=w298:errorcluster)
        n124 = call <vilib>:"Clear Errors.vi"("error in (no error)"=w298) -> ("error out"=w297:errorcluster)  [unwired: 5 in, 1 out]
      }
      frame "프로그램정지" {
        n125 = VISA Close(VISA resource name=w303, error in (no error)=w302) -> (error out=w304:errorcluster)
        n126 = call <vilib>:"Clear Errors.vi"("error in (no error)"=w304) -> ("error out"=w301:errorcluster)  [unwired: 5 in, 1 out]
      }
    }
  }
  n127 = while {
    tunnel: w13 -> [w322]
    shift-right: [w318] -> _
    shift-left: _ -> [w315]
    shift-right: [w317] -> _
    shift-left: _ -> [w314]
    shift-right: [w309] -> _
    shift-left: _ -> [w313]
    shift-right: [w316] -> _
    shift-left: _ -> [w312]
    shift-right: [w311] -> _
    shift-left: -1 -> [w310]
    tunnel: w4 -> [w306]
    stop <- w319 stop-if-true
    # "비전"
    n128 = Dequeue Element(queue=w322, timeout in ms (-1)=w310) -> (queue out=w321:refnum<queue>, element=w323:T2, timed out?=w308:bool, error out=w320:errorcluster)  [unwired: 1 in]
    n129 = case shown="거짓" w308 {
      tunnel: w323 -> [_ w347]
      tunnel: w321 -> [_ w344]
      tunnel: w320 -> [_ w343]
      tunnel: [_ w342] -> w319
      tunnel: [w327 w341] -> w318
      tunnel: [w325 w340] -> w317
      tunnel: [w325 w339] -> w316
      tunnel: [w326 w338] -> w309
      tunnel: w315 -> [w330 w337]
      tunnel: w314 -> [w329 w336]
      tunnel: w313 -> [w328 w335]
      tunnel: w312 -> [_ w334]
      tunnel: [w324 w333] -> w311
      tunnel: w310 -> [w324 w332]
      tunnel: w306 -> [_ w331]
      frame True {
        n130 = call <vilib>:"IMAQdx Snap2.vi"("error in"=w329, "Image In"=w328, "Session In"=w330) -> ("error out"=w325:errorcluster, "Image Out"=w326:T1, "Session Out"=w327:T13)  [unwired: 6 in]
      }
      frame False {
        n131 = Unbundle(w347) -> ("상태"=w346:T14, "값"=w345:variant)
        n132 = case shown="\"닫기\"" w346 {
          tunnel: w345 -> [_ _ _ _ _]
          tunnel: w344 -> [w351 _ _ _ _]
          tunnel: w343 -> [w350 _ _ _ _]
          tunnel: [_ _ _ _ TRUE] -> w342
          tunnel: [_ w358 w368 _ _] -> w341
          tunnel: [_ w357 w367 w374 w383] -> w340
          tunnel: [_ w356 w366 _ _] -> w338
          tunnel: [_ w355 w367 w373 w382] -> w339
          tunnel: w337 -> [_ _ w371 w380 w387]
          tunnel: w336 -> [_ _ w370 w379 w386]
          tunnel: w335 -> [_ _ w369 w378 w385]
          tunnel: w334 -> [_ _ _ w377 w384]
          tunnel: [w349 1000 w372 w381 w390] -> w333
          tunnel: w332 -> [w349 _ w372 w381 w390]
          tunnel: w331 -> [_ _ w361 _ _]
          frame "초기화", Default {
            n133 = Enqueue Element(queue=w351, element=T2 {"상태"=enum."설정", "값"=variant} ("원소"), error in (no error)=w350) -> ()  [unwired: 1 in, 3 out]
          }
          frame "설정" {
            n134 = call <vilib>:"IMAQdx Open Camera.vi"("Session In"=T13 "cam1") -> ("error out"=w357:errorcluster, "Session Out"=w358:T13)  [unwired: 9 in]
            n135 = call "IMAQ Create"("Image Name"="untitled") -> ("New Image"=w356:T1, "error out"=w355:errorcluster)  [unwired: 4 in]
          }
          frame "트리거읽기" {
            w362 = T15 2 items=["사용자 홈"=0, "사용자 데스크탑"=1, "사용자 문서"=2, "사용자 어플리케이션 데이터"=3, "사용자 환경"=4, "사용자 임시"=5, "퍼블릭 문서"=6, "퍼블릭 어플리케이션 데이터"=7, "퍼블릭 환경"=8, "퍼블릭 캐시"=13, "시스템 코어 라이브러리"=9, "시스템 설치된 라이브러리"=10, "어플리케이션 파일"=11, "부팅 볼륨 루트"=12] ("system directory type")
            n136 = Unbundle By Name(w361) -> ("CNN"=w360:refnum<queue>)
            n137 = call <vilib>:"IMAQdx Snap2.vi"("error in"=w370, "Image In"=w369, "Session In"=w371) -> ("error out"=w367:errorcluster, "Image Out"=w366:T1, "Session Out"=w368:T13)  [unwired: 6 in]
            n138 = Enqueue Element(queue=w360, element=T3 {"상태"=enum."CNN 통신", "값"=variant} ("원소")) -> ()  [unwired: 2 in, 3 out]
            n139 = call <vilib>:"Get System Directory.vi"("system directory type"=w362) -> ("system directory"=w365:path)  [unwired: 10 in]
            n140 = Build Path(base path=w365, name or relative path="캡쳐 이미지.jpeg") -> (appended path=w363:path)
            n141 = call-poly "IMAQ Write File 2"("File Path"=w363, "Image"=w366) -> ()  [unwired: 8 in, 2 out]
          }
          frame "닫기" {
            n142 = call <vilib>:"IMAQdx Close Camera.vi"("error in"=w379, "Session In"=w380) -> ("error out"=w376:errorcluster)  [unwired: 9 in]
            n143 = call "IMAQ Dispose"("Image"=w378, "error in (no error)"=w377) -> ("error out"=w375:errorcluster)  [unwired: 4 in]
            n144 = call <vilib>:"Clear Errors.vi"("error in (no error)"=w376) -> ("error out"=w374:errorcluster)  [unwired: 5 in, 1 out]
            n145 = call <vilib>:"Clear Errors.vi"("error in (no error)"=w375) -> ("error out"=w373:errorcluster)  [unwired: 5 in, 1 out]
          }
          frame "프로그램정지" {
            n146 = call <vilib>:"IMAQdx Close Camera.vi"("error in"=w386, "Session In"=w387) -> ("error out"=w389:errorcluster)  [unwired: 9 in]
            n147 = call "IMAQ Dispose"("Image"=w385, "error in (no error)"=w384) -> ("error out"=w388:errorcluster)  [unwired: 4 in]
            n148 = call <vilib>:"Clear Errors.vi"("error in (no error)"=w389) -> ("error out"=w383:errorcluster)  [unwired: 5 in, 1 out]
            n149 = call <vilib>:"Clear Errors.vi"("error in (no error)"=w388) -> ("error out"=w382:errorcluster)  [unwired: 5 in, 1 out]
          }
        }
      }
    }
    "Image" <- w309
    n150 = Wait (ms)(milliseconds to wait=u32 100 ("대기 시간 (ms)")) -> ()  [unwired: 1 out]
  }
  n151 = while {
    tunnel: w6 -> [w397]
    tunnel: w4 -> [w392]
    stop <- w393 stop-if-true
    # "SM(통신)"
    n152 = Dequeue Element(queue=w397) -> (element=w396:T4)  [unwired: 2 in, 3 out]
    n153 = Unbundle(w396) -> ("상태"=w395:enum16{"SM통신", "프로그램정지"}, "값"=w394:variant)
    n154 = case shown="\"프로그램정지\"" w395 {
      tunnel: w394 -> [w422 _]
      tunnel: [_ TRUE] -> w393
      tunnel: w392 -> [w403 _]
      frame "SM통신", Default {
        w418 = path ""  # python X Data
        n155 = Variant To Data(type=dbl[] [], Variant=w422) -> (data=w419:dbl[], error out=w420:errorcluster)  [unwired: 1 in]
        n156 = call-poly <vilib>:"Write Delimited Spreadsheet.vi"("file path (dialog if empty)"=w418, "1D data"=w419, "error in (no error)"=w420) -> ("error out"=w417:errorcluster)  [unwired: 11 in, 1 out]
        n157 = TCP Open Connection(address="localhost" ("주소"), remote port or service name=u16 8103 ("원격 포트 또는 서비스 이름"), error in (no error)=w417) -> (connection ID=w416:refnum<k5>, error out=w415:errorcluster)  [unwired: 2 in]
        n158 = TCP Write(connection ID=w416, data in="Softmax" ("데이터 입력"), error in (no error)=w415) -> (connection ID out=w414:refnum<k5>, error out=w413:errorcluster)  [unwired: 1 in, 1 out]
        n159 = TCP Read(connection ID=w414, bytes to read=9 ("읽을 바이트"), error in (no error)=w413, 7:T16."Immediate" ("모드(standard)")) -> (connection ID out=w412:refnum<k5>, data out=w405:string, error out=w411:errorcluster)  [unwired: 1 in]
        n160 = Decimal String To Number(string=w405) -> (number=w402:i32)  [unwired: 2 in, 1 out]
        n161 = TCP Close Connection(connection ID=w412, error in (no error)=w411) -> ()  [unwired: 1 in, 2 out]
        n162 = Equal?(x=w402, y=6) -> (x = y?=w399:bool)
        n163 = feedback-in #1(w399) -> ()
        n164 = feedback #1() -> (w400:bool)  [unwired: 1 in]
        n165 = Greater?(x=w399, y=w400) -> (0:w398:bool)
        n166 = case shown="1..5" w402 {
          selector: w402 -> [_ w429 _]
          tunnel: ["Normal" w426 "Object Detection" ("문자열")] -> w404
          tunnel: w403 -> [_ w428 w432]
          tunnel: w398 -> [_ _ w433]
          frame 0, Default {
          }
          frame 1..5 {
            n167 = Unbundle By Name(w428) -> ("DB"=w427:refnum<queue>)
            n168 = Decrement(x=w429) -> (x-1=w430:i32)
            n169 = Index Array(array=string[] ["Impact", "X axis F", "X axis B", "Y axis R", "Y axis L"], index=w430) -> (element=w426:string)
            n170 = Bundle By Name(cluster=T7 {"상태"=enum."에러 쓰기", "값"=variant} ("원소"), "값"=w426) -> (w424:T7)
            n171 = Enqueue Element(queue=w427, element=w424) -> ()  [unwired: 2 in, 3 out]
          }
          frame 6 {
            # "물체 감지"
            n172 = case shown="참" w433 {
              tunnel: w432 -> [_ w437]
              frame False {
              }
              frame True {
                n173 = Unbundle By Name(w437) -> ("비전"=w436:refnum<queue>)
                n174 = Enqueue Element(queue=w436, element=T2 {"상태"=enum."트리거읽기", "값"=variant} ("원소")) -> ()  [unwired: 2 in, 3 out]
              }
            }
          }
        }
        "Factory 상태" <- w404
      }
      frame "프로그램정지" {
        n175 = TCP Open Connection(address="localhost" ("주소"), remote port or service name=u16 8103 ("원격 포트 또는 서비스 이름")) -> (connection ID=w449:refnum<k5>, error out=w448:errorcluster)  [unwired: 3 in]
        n176 = TCP Write(connection ID=w449, data in="QUIT" ("데이터 입력"), error in (no error)=w448) -> (connection ID out=w447:refnum<k5>, error out=w446:errorcluster)  [unwired: 1 in, 1 out]
        n177 = TCP Read(connection ID=w447, bytes to read=9 ("읽을 바이트"), error in (no error)=w446, 7:T16."Immediate" ("모드(standard)")) -> (connection ID out=w445:refnum<k5>, error out=w444:errorcluster)  [unwired: 1 in, 1 out]
        n178 = TCP Close Connection(connection ID=w445, error in (no error)=w444) -> ()  [unwired: 1 in, 2 out]
      }
    }
  }
  n179 = while {
    tunnel: w5 -> [w454]
    tunnel: w4 -> [w451]
    stop <- w450 stop-if-true
    # "CNN(통신1)"
    n180 = Dequeue Element(queue=w454) -> (element=w455:T3)  [unwired: 2 in, 3 out]
    n181 = Unbundle(w455) -> ("상태"=w453:enum16{"CNN 통신", "프로그램정지"}, "값"=w452:variant)
    n182 = case shown="\"프로그램정지\"" w453 {
      tunnel: w452 -> [_ _]
      tunnel: w451 -> [w460 _]
      tunnel: [_ TRUE] -> w450
      frame "CNN 통신", Default {
        n183 = for {
          tunnel: string[] ["SHAPE", "COLOR"] -> [w465] mode=indexing
          tunnel: [w462] -> w457 mode=indexing
          n184 = TCP Open Connection(address="localhost" ("주소"), remote port or service name=u16 8104 ("원격 포트 또는 서비스 이름")) -> (connection ID=w472:refnum<k5>, error out=w471:errorcluster)  [unwired: 3 in]
          n185 = TCP Write(connection ID=w472, data in=w465, error in (no error)=w471) -> (connection ID out=w470:refnum<k5>, error out=w469:errorcluster)  [unwired: 1 in, 1 out]
          n186 = TCP Read(connection ID=w470, bytes to read=9 ("읽을 바이트"), error in (no error)=w469, 7:T16."Immediate" ("모드(standard)")) -> (connection ID out=w468:refnum<k5>, data out=w462:string, error out=w467:errorcluster)  [unwired: 1 in]
          n187 = TCP Close Connection(connection ID=w468, error in (no error)=w467) -> ()  [unwired: 1 in, 2 out]
        }
        "CNN Result" <- w457
        n188 = Unbundle By Name(w460) -> ("DB"=w459:refnum<queue>)
        n189 = Bundle By Name(cluster=T7 {"상태"=enum."초기화", "값"=variant} ("원소"), "값"=w457) -> (w456:T7)
        n190 = Enqueue Element(queue=w459, element=w456) -> ()  [unwired: 2 in, 3 out]
      }
      frame "프로그램정지" {
        n191 = TCP Open Connection(address="localhost" ("주소"), remote port or service name=u16 8104 ("원격 포트 또는 서비스 이름")) -> (connection ID=w485:refnum<k5>, error out=w484:errorcluster)  [unwired: 3 in]
        n192 = TCP Write(connection ID=w485, data in="QUIT" ("데이터 입력"), error in (no error)=w484) -> (connection ID out=w483:refnum<k5>, error out=w482:errorcluster)  [unwired: 1 in, 1 out]
        n193 = TCP Read(connection ID=w483, bytes to read=9 ("읽을 바이트"), error in (no error)=w482, 7:T16."Immediate" ("모드(standard)")) -> (connection ID out=w481:refnum<k5>, error out=w480:errorcluster)  [unwired: 1 in, 1 out]
        n194 = TCP Close Connection(connection ID=w481, error in (no error)=w480) -> ()  [unwired: 1 in, 2 out]
      }
    }
  }
